vi "bluetoothTest.vi"() -> ()   [LabVIEW 2015]
uses:
  <vilib>/myRIO/Instrument Drivers/Onboard IO/UART/typedef/VISA Configuration.ctl
  <vilib>/Instr/_visa.llb/VISA Configure Serial Port (Instr).vi
  <vilib>/myRIO/Express VI/Onboard IO/UART/UART Express VI.xnode
  <vilib>/myRIO/Instrument Drivers/Onboard IO/UART/UART.lvlib
panel:
  out "trimmed string 2":string
  out "Waveform Chart 2":i32(graph)
  out "trimmed string":string
  out "Numeric 2":dbl
  out "Waveform Chart":i32(graph)
  out "match + rest of string":string
  out "Numeric":i32
  out "substring before match 2":string
  in  "stop":bool
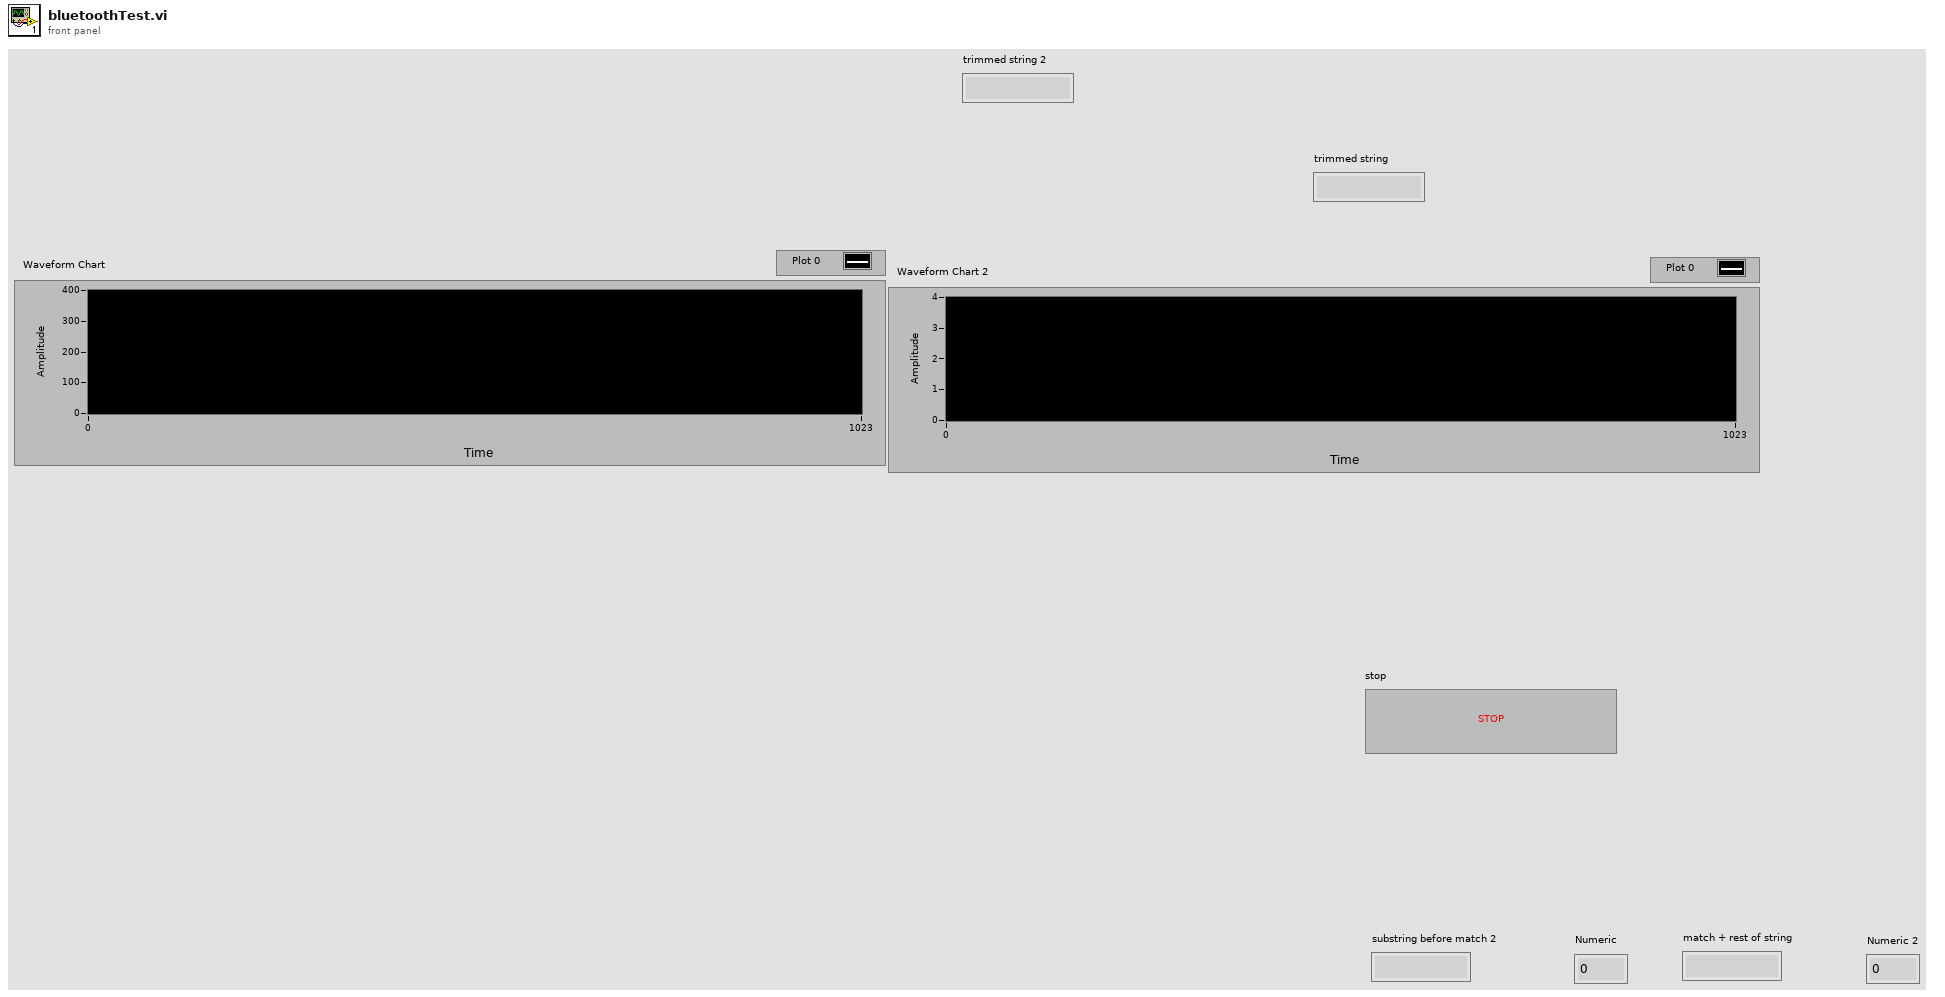
[diagram p1: front panel]
types:
  T1 = typedef "UART.lvlib/VISA Configuration.ctl" = cluster{"baud rate (9600)":u32, "data bits (8)":u16, "parity (0:none)":enum16{"None", "Odd", "Even", "Mark", "Space"}, "stop bits (10: 1 bit)":u16, "flow control (0:none)":u16, "termination char\n(0xA = '\\n' = LF) ":u8, "Enable Termination\nChar (T)":bool, "timeout (10sec)":u32}
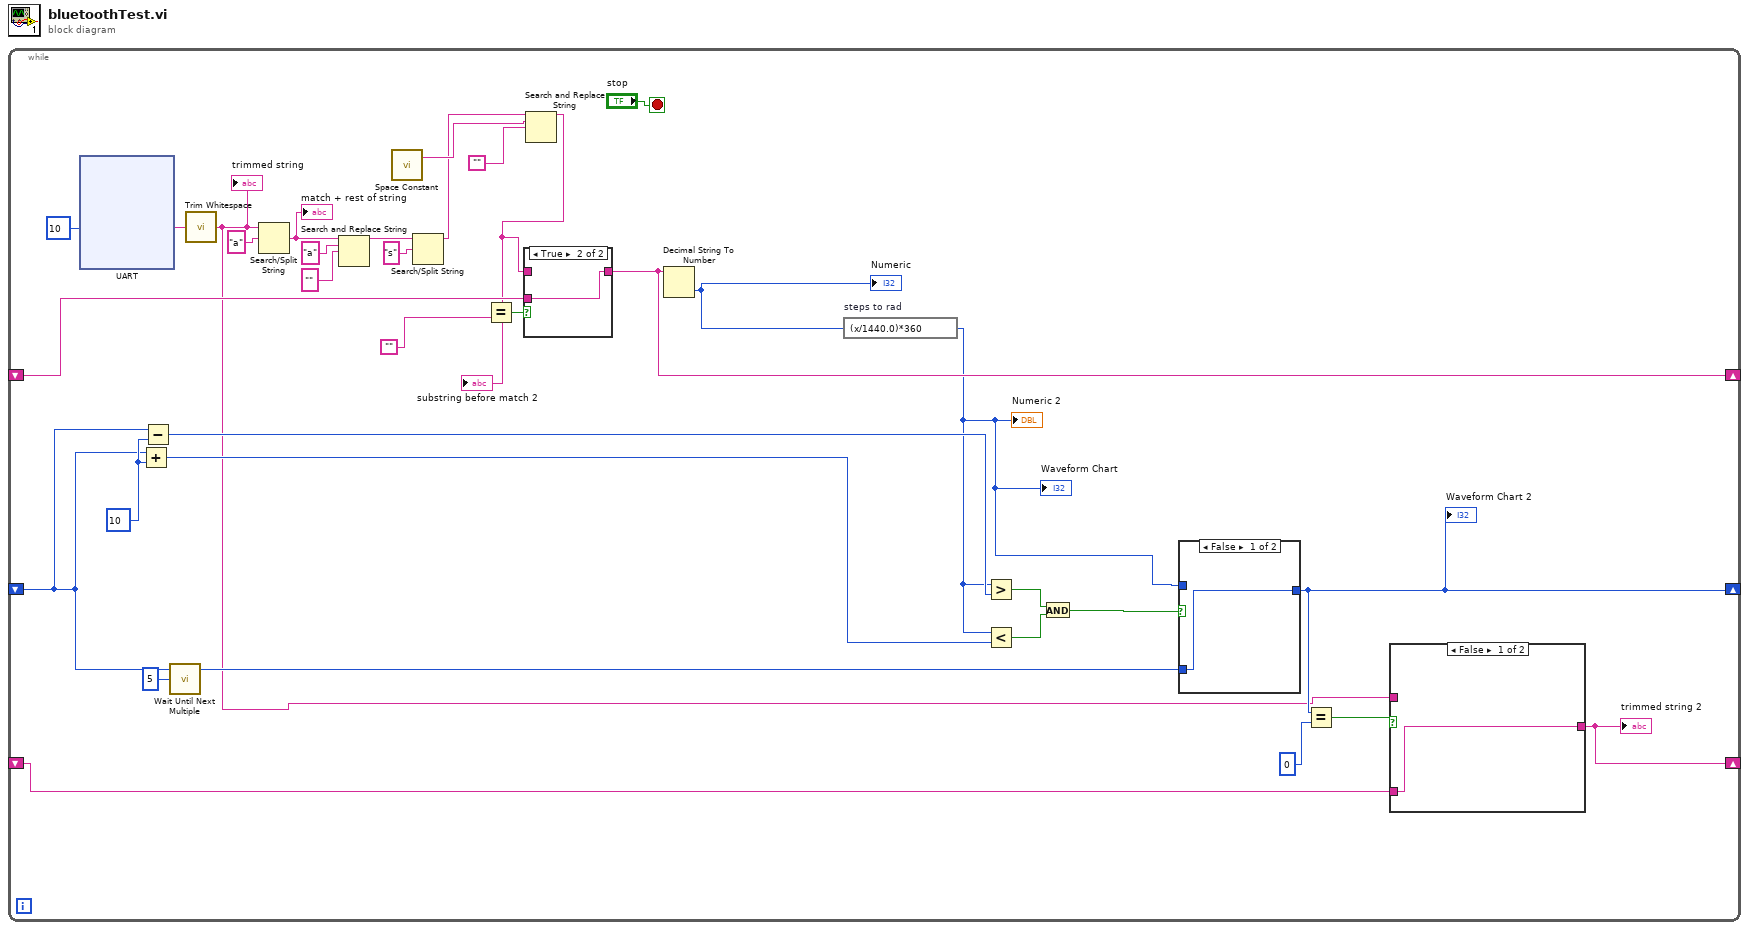
[diagram p0: block diagram]
diagram:
  n1 = while {
    shift-right: [w24] -> _
    shift-left: _ -> [w23]
    shift-right: [w12] -> _
    shift-left: _ -> [w14]
    shift-right: [w8] -> _
    shift-left: _ -> [w7]
    stop <- "stop" stop-if-true
    w21 = 10 ("y")
    n2 = xnode "UART"("Character Count"=u32 10) -> ("Characters Read"=w29:string)  [unwired: 1 in, 1 out]
    n3 = Add(x=w14, y=w21) -> (x+y=w18:i32)
    n4 = Subtract(x=w14, y=w21) -> (x-y=w17:i32)
    n5 = call "Wait Until Next Multiple"("Count(mSec)"=u32 5) -> ()  [unwired: 1 out]
    n6 = call <vilib>:"Trim Whitespace.vi"("string"=w29) -> ("trimmed string"=w9:string)  [unwired: 1 in]
    "trimmed string" <- w9
    n7 = Search/Split String(string=w9, search string/char (-)="a") -> (match + rest of string=w28:string)  [unwired: 1 in, 2 out]
    "match + rest of string" <- w28
    n8 = Search and Replace String(input string=w28, search string="a", replace string="" ("replace string (\"\")")) -> (result string=w27:string)  [unwired: 5 in, 3 out]
    n9 = call <vilib>:"Space Constant.vi"() -> ("String"=w3:string)
    n10 = Search/Split String(string=w27, search string/char (-)="s") -> (substring before match=w2:string)  [unwired: 1 in, 2 out]
    n11 = Search and Replace String(input string=w2, search string=w3, replace string="") -> (result string=w1:string)  [unwired: 5 in, 3 out]
    "substring before match 2" <- w1
    n12 = Equal?(x=w1, y="") -> (x = y?=w30:bool)
    n13 = case shown="True" w30 {
      tunnel: w1 -> [w38 _]
      tunnel: w23 -> [_ w39]
      tunnel: [w38 w39] -> w24
      frame False {
      }
      frame True {
      }
    }
    n14 = Decimal String To Number(string=w24) -> (number=w13:i32)  [unwired: 2 in, 1 out]
    "Numeric" <- w13
    n15 = expression code="(x/1440.0)*360" "steps to rad"(w13) -> (w15:i32)
    "Waveform Chart" <- w15
    "Numeric 2" <- w15
    n16 = Greater?(x=w15, y=w17) -> (0:w20:bool)
    n17 = Less?(x=w15, y=w18) -> (x < y?=w19:bool)
    n18 = And(x=w20, y=w19) -> (x .and. y?=w16:bool)
    n19 = case shown="False" w16 {
      tunnel: w15 -> [_ w37]
      tunnel: [w36 w37] -> w12
      tunnel: w14 -> [w36 _]
      frame False {
      }
      frame True {
      }
    }
    "Waveform Chart 2" <- w12
    n20 = Equal?(x=w12, y=0) -> (x = y?=w10:bool)
    n21 = case shown="False" w10 {
      tunnel: [w34 w35] -> w8
      tunnel: w9 -> [_ w35]
      tunnel: w7 -> [w34 _]
      frame False {
      }
      frame True {
      }
    }
    "trimmed string 2" <- w8
  }
